vi "TCP_connection.vi"() -> ()   [LabVIEW 2020]
uses:
  <vilib>/Utility/error.llb/DialogType.ctl
panel:
  out "Iterative Results":T1(array[cluster])
  in  "PortName":string="localhost"
  in  "PortNumber":u16=62358
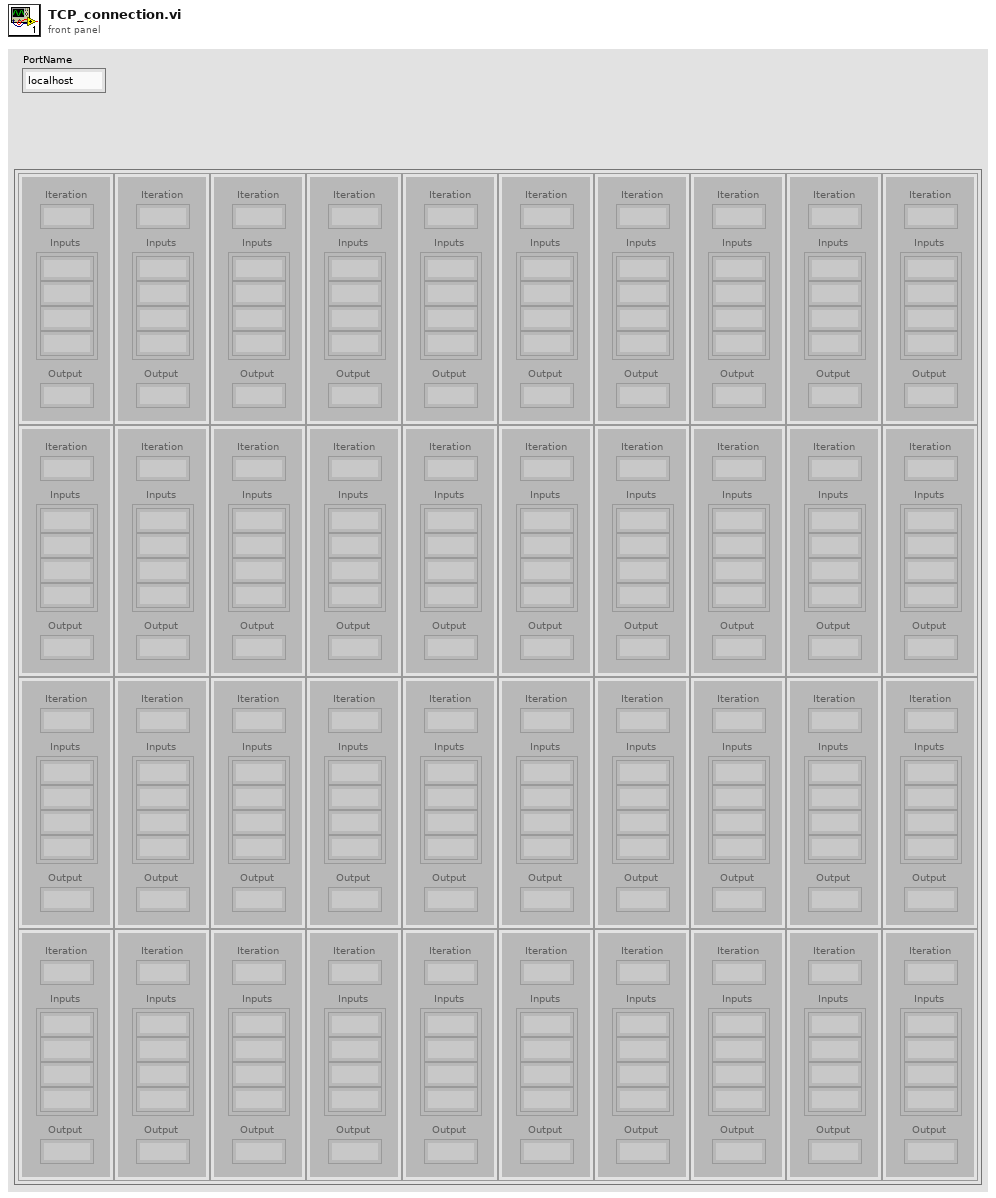
[diagram p1: front panel]
types:
  T1 = cluster{"Iteration":i32, "Inputs":dbl[], "Output":dbl}[][]
  T2 = typedef "DialogType.ctl" = u16
  T3 = cluster{"Iteration":i32, "Inputs":dbl[], "Output":dbl}
  T4 = enum16{"Standard", "Buffered", "CRLF", "Immediate"}
  T5 = cluster{"Iteration":i32, "Inputs":dbl[], "Output":dbl}[]
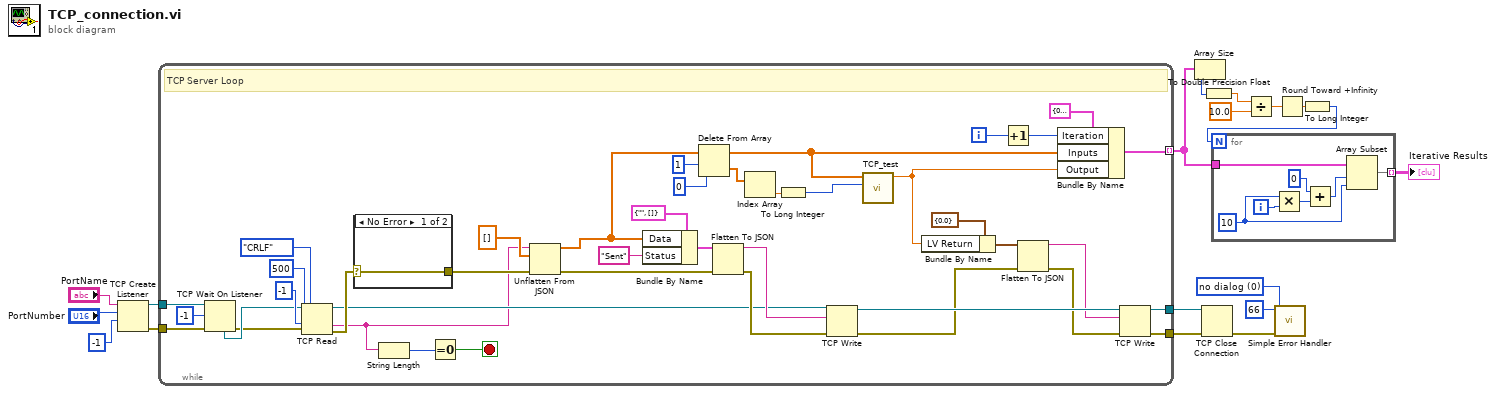
[diagram p0: block diagram]
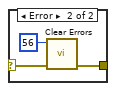
[diagram p2: hidden frame]
diagram:
  w11 = T2 0 items=["no dialog", "OK message", "continue or stop message", "OK message + warnings", "continue/stop + warnings"] ("type of dialog (OK msg:1)")
  n1 = TCP Create Listener(9:-1 ("timeout ms (25000)"), 10:"PortNumber", 11:"PortName") -> (0:w1:errorcluster, 3:w2:refnum<k5>)  [unwired: 2 in, 1 out]
  n2 = while {
    tunnel: [w40] -> w15
    tunnel: [w38] -> w13
    tunnel: [w34] -> w10 mode=indexing
    tunnel: w2 -> [w26]
    tunnel: w1 -> [w24]
    i -> [w36]
    stop <- w55 stop-if-true
    # "TCP Server Loop"
    n3 = TCP Wait On Listener(8:w24, 9:-1 ("timeout ms (wait forever: -1)"), 11:w26) -> (0:w23:errorcluster, 4:w25:refnum<k5>)  [unwired: 1 in, 3 out]
    n4 = TCP Read(connection ID=w25, bytes to read=500, error in (no error)=w23, 7:T4."CRLF" ("mode (standard)"), 9:-1 ("timeout ms (25000)")) -> (connection ID out=w39:refnum<k5>, data out=w22:string, error out=w42:errorcluster)
    n5 = case shown="No Error" w42 {
      selector: w42 -> [w60 w62]
      tunnel: [w60 w63] -> w41
      frame No Error {
      }
      frame Error {
        n6 = call <vilib>:"Clear Errors.vi"("error in (no error)"=w62, "specific error code to clear (0: all)"=56) -> ("error out"=w63:errorcluster)  [unwired: 4 in, 1 out]
      }
    }
    n7 = String Length(string=w22) -> (length=w56:i32)
    n8 = Equal To 0?(x=w56) -> (x = 0?=w55:bool)
    n9 = Unflatten From JSON(JSON string=w22, type and defaults=dbl[] [], error in (no error)=w41) -> (value=w29:dbl[], error out=w54:errorcluster)  [unwired: 4 in]
    n10 = Bundle By Name(cluster=cluster{"Status":string, "Data":dbl[]} {"Status"="", "Data"=[]}, "Data"=w29, "Status"="Sent") -> (w50:cluster{"Status":string, "Data":dbl[]})
    n11 = Delete From Array(array=w29, length=1, index=0) -> (deleted portion=w30:dbl[], array with subset deleted=w20:dbl[])
    n12 = Flatten To JSON(anything=w50, error in (no error)=w54) -> (JSON string=w45:string, 11:w53:errorcluster)  [unwired: 1 in]
    n13 = Index Array(array=w30) -> (element=w28:dbl)  [unwired: 1 in]
    n14 = To Long Integer(number=w28) -> (32bit integer=w19:i32)
    n15 = TCP Write(connection ID=w39, data in=w45, error in (no error)=w53) -> (connection ID out=w49:refnum<k5>, error out=w48:errorcluster)  [unwired: 1 in, 1 out]
    n16 = call "TCP_test.vi"("Mode"=w19, "Array"=w20) -> ("Numeric"=w21:dbl)  [unwired: 9 in]
    n17 = Bundle By Name(cluster=cluster{"LV Return":dbl} {"LV Return"=0.0}, "LV Return"=w21) -> (w44:cluster{"LV Return":dbl})
    n18 = Increment(x=w36) -> (x+1=w35:i32)
    n19 = Flatten To JSON(anything=w44, error in (no error)=w48) -> (JSON string=w46:string, 11:w47:errorcluster)  [unwired: 1 in]
    n20 = Bundle By Name(cluster=T3 {"Iteration"=0, "Inputs"=[], "Output"=0.0}, "Iteration"=w35, "Inputs"=w20, "Output"=w21) -> (w34:T3)
    n21 = TCP Write(connection ID=w49, data in=w46, error in (no error)=w47) -> (connection ID out=w40:refnum<k5>, error out=w38:errorcluster)  [unwired: 1 in, 1 out]
  }
  n22 = Array Size(array=w10) -> (size(s)=w7:i32)
  n23 = TCP Close Connection(connection ID=w15, error in (no error)=w13) -> (error out=w14:errorcluster)  [unwired: 2 out]
  n24 = To Double Precision Float(number=w7) -> (double precision float=w6:dbl)
  n25 = Divide(x=w6, y=10.0) -> (x/y=w9:dbl)
  n26 = call <vilib>:"Simple Error Handler.vi"("error code (no error:0)"=66, "type of dialog (OK msg:1)"=w11, "error in (no error)"=w14) -> ()  [unwired: 7 out]
  n27 = Round Toward +Infinity(x=w9) -> (ceil(x): smallest int >= x=w5:dbl)
  n28 = To Long Integer(number=w5) -> (32bit integer=w4:i32)
  n29 = for {
    N: w4 -> [_]
    tunnel: w10 -> [w70]
    tunnel: [w64] -> w3 mode=indexing
    i -> [w69]
    w68 = 10 ("length")
    n30 = Multiply(x=w68, y=w69) -> (x*y=w67:i32)
    n31 = Add(x=0 ("index"), y=w67) -> (x+y=w65:i32)
    n32 = Array Subset(array=w70, index=w65, length=w68) -> (w64:T5)
  }
  "Iterative Results" <- w3
